vi "1D linear array generator_dataview.vi"(1 "step X":sgl=3.0 format="%.3f", 2 "initial X":sgl=0.01 format="%.2f", 3 "final X":sgl=7.0 format="%.2f") -> (0 "Array":dbl[](array[numeric]))   [LabVIEW 2019]
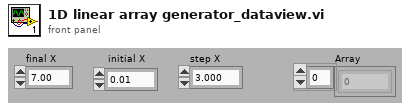
[diagram p1: front panel]
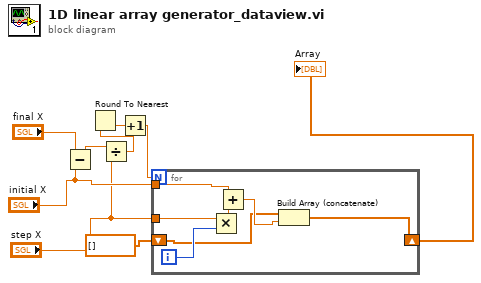
[diagram p0: block diagram]
diagram:
  n1 = Subtract(x="final X", y="initial X") -> (x-y=w2:sgl)
  n2 = Divide(x=w2, y="step X") -> (x/y=w6:sgl)
  n3 = Round To Nearest(number=w6) -> (nearest integer value=w3:sgl)
  n4 = Increment(x=w3) -> (x+1=w7:sgl)
  n5 = for {
    N: w7 -> [_]
    tunnel: "step X" -> [w14]
    tunnel: "initial X" -> [w13]
    shift-right: [w11] -> w9
    shift-left: dbl[] [] -> [w10]
    i -> [w15]
    n6 = Multiply(x=w14, y=w15) -> (x*y=w16:sgl)
    n7 = Add(x=w13, y=w16) -> (x+y=w12:sgl)
    n8 = Build Array (concatenate)(w10, w12) -> (w11:dbl[])
  }
  "Array" <- w9
